vi "Register Cluster.vi"(7 "Package Name":string, 8 "error in":errorcluster, 10 "Cluster":variant, 11 "gRPCid in":T1) -> (0 "error out":errorcluster, 3 "gRPCid out":T1)   [LabVIEW 2019, in "grpc-lvsupport.lvlib"]
uses:
  grpc-lvsupport.lvlib
  Shared/grpcId.ctl
  <vilib>/Utility/error.llb/Error Cluster From Error Code.vi
  <resource>/labview_grpc_server.dll
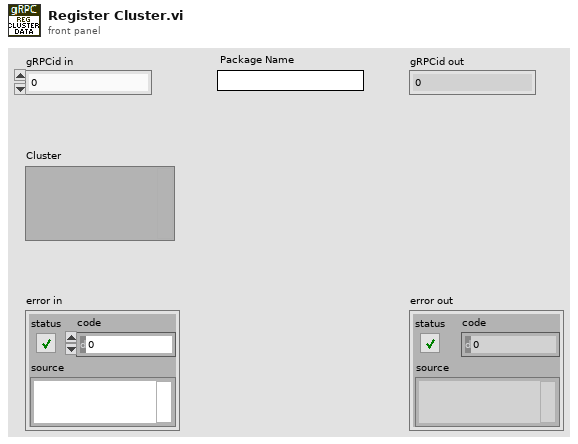
[diagram p1: front panel]
types:
  T1 = typedef "grpc-lvsupport.lvlib/grpcId.ctl" = u64
  T2 = typedef "grpc-lvsupport.lvlib/Message Metadata.ctl" = cluster{"Version":i32, "Name":string, "Type Url":string, "Elements":T3[], "Has Oneof":bool}
  T3 = typedef "grpc-lvsupport.lvlib/Message Element Metadata.ctl" = cluster{"Field Name":string, "Embedded Message Name":string, "Protobuf Index":i32, "MessageElementType":T4, "Repeated":bool, "Is in Oneof":bool, "Oneof Container Name":string}
  T4 = typedef "grpc-lvsupport.lvlib/Message Element Type.ctl" = enum32{"Int32Value", "FloatValue", "DoubleValue", "BoolValue", "StringValue", "MessageValue", "Int64Value", "UInt32Value", "UInt64Value", "EnumValue", "Bytes", "Fixed64", "Fixed32", "SFixed64", "SFixed32", "SInt64", "SInt32"}
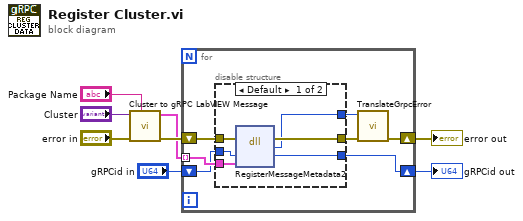
[diagram p0: block diagram]
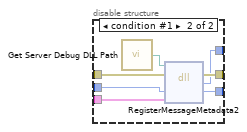
[diagram p2: hidden frame]
diagram:
  n1 = call "Cluster to gRPC LabVIEW Message.vi"("Package Name"="Package Name", "error in"="error in", "Cluster"="Cluster") -> ("error out"=w8:errorcluster, "gRPC Message Metadata []"=w5:T2[])  [unwired: 6 in, 1 out]
  n2 = for {
    tunnel: w5 -> [w13] mode=indexing
    shift-right: [w11] -> w6
    shift-left: "gRPCid in" -> [w12]
    shift-right: [w10] -> w1
    shift-left: w8 -> [w15]
    n3 = disable-structure shown="Default" {
      disable-tunnel: w15 -> [w21 w28]
      disable-tunnel: [w20 w27] -> w14
      disable-tunnel: w13 -> [w19 w26]
      disable-tunnel: w12 -> [w18 w25]
      disable-tunnel: [w17 w24] -> w11
      disable-tunnel: [w16 w23] -> w9
      frame condition #0 (active) {
        n4 = dll-call lib="C:/Program Files (x86)/National Instruments/LabVIEW 2024/resource/labview_grpc_server.*" fn="RegisterMessageMetadata2"(error in=w21, "serverId"=w18, "metadata"=w19) -> (error out=w20:errorcluster, "return type"=w16:i32, "serverId"=w17:T1)  [unwired: 3 in, 1 out]
      }
      frame condition #1 {
        n5 = call "Get Server Debug DLL Path.vi"() -> ("DLL Path"=w22:path)
        n6 = dll-call lib="?" fn="RegisterMessageMetadata2"(path in=w22, error in=w28, "serverId"=w25, "metadata"=w26) -> (error out=w27:errorcluster, "return type"=w23:i32, "serverId"=w24:T1)  [unwired: 2 in, 1 out]
      }
    }
    n7 = call "TranslateGrpcError.vi"("error in"=w14, "Error Code"=w9) -> ("error out"=w10:errorcluster)  [unwired: 9 in]
  }
  "error out" <- w1
  "gRPCid out" <- w6
